vi "Design N FIR filters.vi"(4 "arrOptionalFilterSpecs":T2(array[cluster]) {"SB Gain" format="%0.2f"; "PB Gain" format="%0.2f"}, 6 "arrFilterSpecs":T1(array[cluster]) {"Lower SB" format="%0.2p"; "Upper SB" format="%0.2p"; "Lower PB" format="%0.2p"; "Upper PB" format="%0.2p"}, 7 "redesign filters":bool[](array[boolean]), 8 "error in":errorcluster, 11 "arrdt":dbl[](array[numeric]) format="%0.2f") -> (0 "error out":errorcluster, 1 "arrForward Coefficients":dbl[][](array[numeric]) format="%0.2f", 3 "arrFilterInfo":T3(array[cluster]) {"phase H(w)"."df" format="%0.2f"; "phase H(w)"."f0" format="%0.2f"; "phase H(w)"."Phase H(w)" format="%0.2f"; "magnitude H(w)"."df" format="%0.2f"; "magnitude H(w)"."f0" format="%0.2f"; "magnitude H(w)"."Mag H(w)" format="%0.2f"}, 5 "reset filter states":bool[](array[boolean]))   [LabVIEW 2020, in "NI_MAPro.lvlib"]
uses:
  NI_MAPro.lvlib
  NI_MABase.lvlib
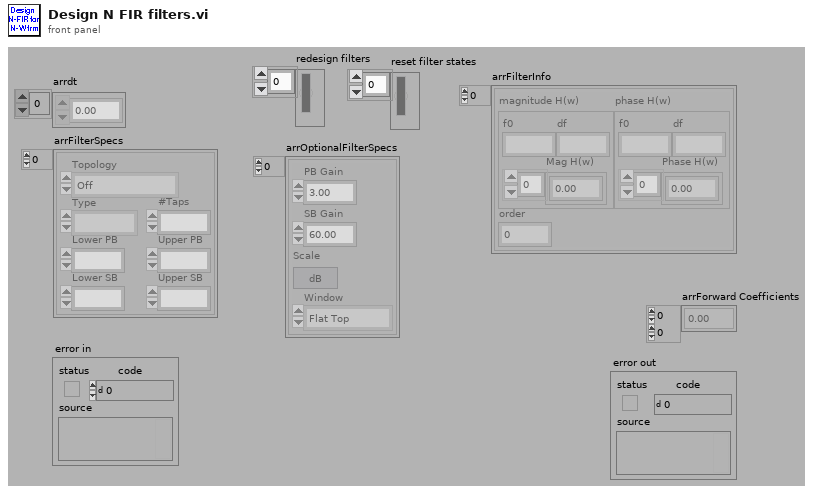
[diagram p1: front panel]
types:
  T1 = cluster{"Topology":enum16{"Off", "FIR by Specification", "Equi-ripple FIR", "Windowed FIR"}, "Type":enum16{"Lowpass", "Highpass", "Bandpass", "Bandstop"}, "#Taps":i32, "Lower PB":dbl, "Upper PB":dbl, "Lower SB":dbl, "Upper SB":dbl}[]
  T2 = cluster{"PB Gain":dbl, "SB Gain":dbl, "Scale":bool, "Window":enum16{"None", "Hanning", "Hamming", "Triangular", "Blackman", "Exact Blackman", "Blackman-Harris", "Kaiser-Bessel", "Flat Top"}}[]
  T3 = cluster{"magnitude H(w)":cluster{"f0":dbl, "df":dbl, "Mag H(w)":dbl[]}, "phase H(w)":cluster{"f0":dbl, "df":dbl, "Phase H(w)":dbl[]}, "order":i32}[]
  T4 = cluster{"PB Gain":dbl, "SB Gain":dbl, "Scale":bool, "Window":enum16{"None", "Hanning", "Hamming", "Triangular", "Blackman", "Exact Blackman", "Blackman-Harris", "Kaiser-Bessel", "Flat Top"}}
  T5 = cluster{"magnitude H(w)":cluster{"f0":dbl, "df":dbl, "Mag H(w)":dbl[]}, "phase H(w)":cluster{"f0":dbl, "df":dbl, "Phase H(w)":dbl[]}, "order":i32}
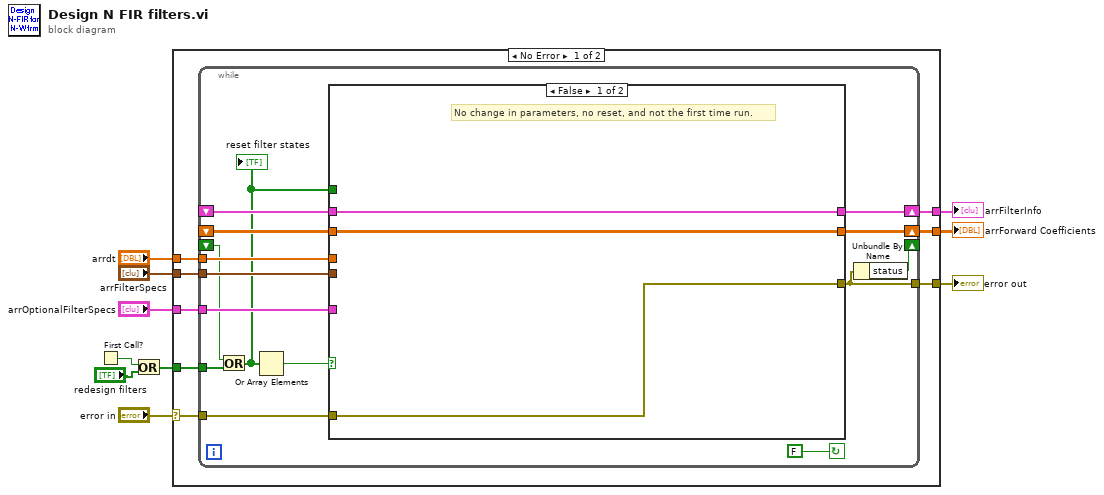
[diagram p0: block diagram]
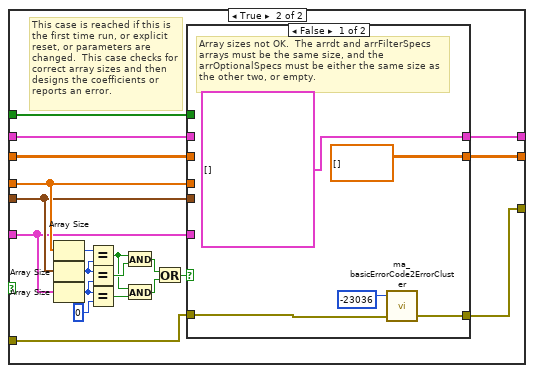
[diagram p2: hidden frame]
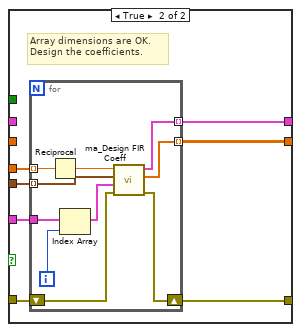
[diagram p3: hidden frame]
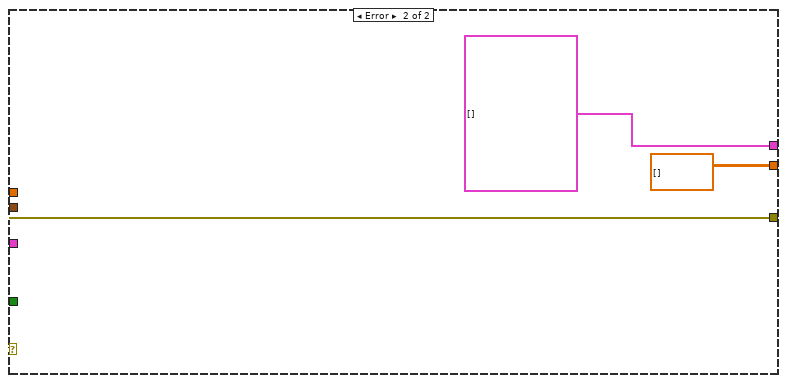
[diagram p4: hidden frame]
diagram:
  n1 = First Call?() -> (First Call?: T/F=w3:bool)
  n2 = Or(x=w3, y="redesign filters") -> (x .or. y?=w1:bool[])
  n3 = case shown="No Error" "error in" {
    selector: "error in" -> [w17 w81]
    tunnel: [w18 w81] -> w10
    tunnel: "arrOptionalFilterSpecs" -> [w16 _]
    tunnel: "arrFilterSpecs" -> [w15 _]
    tunnel: "arrdt" -> [w14 _]
    tunnel: [w13 dbl[][] [] ("Forward Coefficients")] -> w5
    tunnel: [w12 T3 []] -> w4
    tunnel: w1 -> [w11 _]
    frame No Error {
      n4 = while {
        tunnel: w11 -> [w21]
        tunnel: w14 -> [w26]
        tunnel: w15 -> [w28]
        tunnel: w16 -> [w27]
        tunnel: w17 -> [w25]
        tunnel: [w24] -> w18
        shift-left: _ -> [w30]
        shift-right: [w31] -> w12
        shift-left: _ -> [w33]
        shift-right: [w29] -> w13
        shift-right: [w23] -> _
        shift-left: _ -> [w22]
        stop <- FALSE continue-if-true
        n5 = Or(x=w22, y=w21) -> (x .or. y?=w20:bool[])
        "reset filter states" <- w20
        n6 = Or Array Elements(Boolean array=w20) -> (logical OR=w19:bool)
        n7 = case shown="False" w19 {
          tunnel: w33 -> [w36 w39]
          tunnel: [w35 w56] -> w31
          tunnel: w30 -> [w35 w37]
          tunnel: [w36 w55] -> w29
          tunnel: [w34 w54] -> w24
          tunnel: w26 -> [_ w44]
          tunnel: w28 -> [_ w43]
          tunnel: w27 -> [_ w42]
          tunnel: w25 -> [w34 w40]
          tunnel: w20 -> [_ w38]
          frame False {
            # "No change in parameters, no reset, and not the first time run."
          }
          frame True {
            # "This case is reached if this is the first time run, or explicit reset, or parameters are changed.  This case checks for correct array sizes and then designs the coefficients or reports an error."
            n8 = Array Size(array=w44) -> (size(s)=w53:i32)
            n9 = Array Size(array=w43) -> (size(s)=w52:i32)
            n10 = Array Size(array=w42) -> (size(s)=w50:i32)
            n11 = Equal?(x=w53, y=w52) -> (x = y?=w47:bool)
            n12 = Equal?(x=w52, y=w50) -> (x = y?=w51:bool)
            n13 = Equal?(x=w50, y=0) -> (x = y?=w48:bool)
            n14 = And(x=w47, y=w51) -> (x .and. y?=w46:bool)
            n15 = And(x=w47, y=w48) -> (x .and. y?=w45:bool)
            n16 = Or(x=w46, y=w45) -> (x .or. y?=w41:bool)
            n17 = case shown="False" w41 {
              tunnel: [T3 [] w68] -> w56
              tunnel: [dbl[][] [] ("Forward Coefficients") w67] -> w55
              tunnel: [w59 w66] -> w54
              tunnel: w44 -> [_ w65]
              tunnel: w43 -> [_ w64]
              tunnel: w42 -> [_ w63]
              tunnel: w40 -> [w58 w62]
              tunnel: w39 -> [_ _]
              tunnel: w38 -> [_ _]
              tunnel: w37 -> [_ _]
              frame False {
                # "Array sizes not OK.  The arrdt and arrFilterSpecs arrays must be the same size, and the arrOptionalSpecs must be either the same size as the other two, or empty."
                n18 = call "ma_basicErrorCode2ErrorCluster.vi"("error in (no error)"=w58, "Error Code"=-23036) -> ("error out"=w59:errorcluster)  [unwired: 1 in]
              }
              frame True {
                # "Array dimensions are OK.  \nDesign the coefficients."
                n19 = for {
                  tunnel: w64 -> [w71] mode=indexing
                  tunnel: [w78] -> w67 mode=indexing
                  tunnel: w63 -> [w77]
                  tunnel: w65 -> [w72] mode=indexing
                  tunnel: [w75] -> w68 mode=indexing
                  shift-right: [w74] -> w66
                  shift-left: w62 -> [w73]
                  i -> [w76]
                  n20 = Reciprocal(x=w72) -> (1/x=w70:dbl)
                  n21 = Index Array(array=w77, index=w76) -> (element=w69:T4)
                  n22 = call "ma_Design FIR Coeff.vi"("error in"=w73, "Optional FIR Filter Specifications"=w69, "FIR Filter Specifications"=w71, "Sampling Frequency"=w70) -> ("error out"=w74:errorcluster, "Forward Coefficients"=w78:dbl[], "Filter Information"=w75:T5)  [unwired: 5 in]
                }
              }
            }
          }
        }
        n23 = Unbundle By Name(w24) -> ("status"=w23:bool)
      }
    }
    frame Error {
    }
  }
  "error out" <- w10
  "arrForward Coefficients" <- w5
  "arrFilterInfo" <- w4
